vi "FOC Algorithm.vi"() -> ()   [LabVIEW 2025]
panel:
  in  "Speed Setpoint":fxp<+/-,32,16>=500.0
  in  "Kp (speed)":fxp<+,32,8>=1.2099742889404297e-05
  in  "Ki (speed)":fxp<+,32,8>=4.76837158203125e-07
  in  "PWM  Period (T)":fxp<+,32,10>=512.0
  in  "Kp (Id)":fxp<+/-,32,4>=0.6000000014901161
  in  "Ki (Id)":fxp<+/-,32,4>=0.3999999985098839
  in  "Kp (Iq)":fxp<+/-,32,8>=0.550000011920929
  in  "Ki (Iq)":fxp<+/-,32,8>=0.30000001192092896
  out "Id":fxp<+/-,32,4> format="%.6e"
  out "Iq":fxp<+/-,32,4> format="%.6e"
  out "Va":fxp<+/-,37,17> format="%.5e"
  out "Vb":fxp<+/-,37,17> format="%.5e"
  out "Vc":fxp<+/-,37,17> format="%.5e"
  in  "1/Vdc":fxp<+/-,32,16>=512.0
  out "PWM1":fxp<+,16,16>
  out "PWM2":fxp<+,16,16>
  out "PWM3":fxp<+,16,16>
  out "Vq":fxp<+/-,37,17> format="%.5e"
  out "Vd":fxp<+/-,32,4> format="%.5e"
  out "Valpha":fxp<+/-,32,12> format="%.8g"
  out "Vbeta":fxp<+/-,32,12> format="%.8g"
  out "Speed PI Output":fxp<+,32,9> format="%.8g"
  out "Ta":fxp<+/-,37,17> format="%.8g"
  out "Tb":fxp<+/-,37,17> format="%.8g"
  out "Tc":fxp<+/-,37,17> format="%.8g"
  in  "RPM":fxp<+/-,32,16>
  in  "Ia":fxp<+/-,32,4> format="%#_8g"
  in  "Ib":fxp<+/-,32,4> format="%.8g"
  in  "Theta":fxp<+/-,32,16> format="%.8g"
  in  "stop":bool
  # "Control Inputs"
  # "Control Gains"
  # "Control Constants"
  # "Calculated Values and PWM Output"
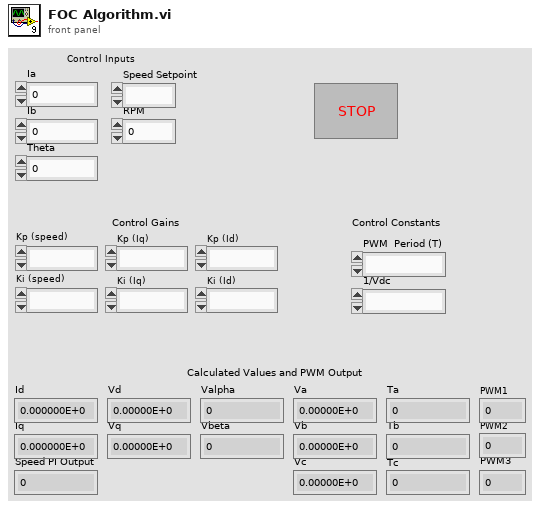
[diagram p1: front panel]
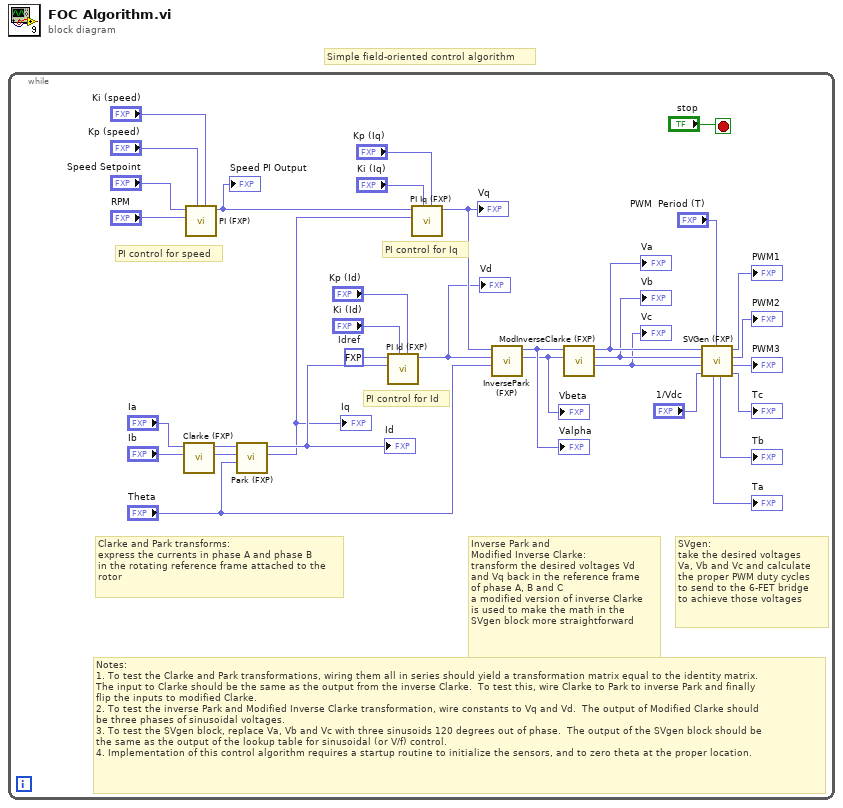
[diagram p0: block diagram]
diagram:
  # "Simple field-oriented control algorithm"
  n1 = while {
    stop <- "stop" stop-if-true
    w28 = fxp<+/-,32,1> 0.0  # Idref
    # "Notes:\n1. To test the Clarke and Park transformations, wiring them all in series should yield a transformation matrix equal to the identity matrix.\nThe input to Clarke should be the same as the output from the inverse Clarke.  To test this, wire Clarke to Park to inverse Park and finally\nflip the inputs to modified Clarke.\n2. To test the inverse Park and Modified Inverse Clarke transformation, wire constants to Vq and Vd.  The output of Modified Clarke should \nbe three phases of sinusoidal voltages.\n3. To test the SVgen block, replace Va, Vb and Vc with three sinusoids 120 degrees out of phase.  The output of the SVgen block should be\nthe same as the output of the lookup table for sinusoidal (or V/f) control.\n4. Implementation of this control algorithm requires a startup routine to initialize the sensors, and to zero theta at the proper location."
    # "SVgen:\ntake the desired voltages\nVa, Vb and Vc and calculate\nthe proper PWM duty cycles\nto send to the 6-FET bridge\nto achieve those voltages"
    # "Inverse Park and \nModified Inverse Clarke:\ntransform the desired voltages Vd\nand Vq back in the reference frame\nof phase A, B and C\na modified version of inverse Clarke\nis used to make the math in the \nSVgen block more straightforward"
    # "Clarke and Park transforms:\nexpress the currents in phase A and phase B\nin the rotating reference frame attached to the\nrotor"
    # "PI control for Id"
    # "PI control for Iq"
    # "PI control for speed"
    n2 = call "Clarke (FXP).vi"("B"="Ib", "A"="Ia") -> ("x*y"=w23:fxp<+/-,32,5>, "A"=w22:fxp<+/-,32,5>)  [unwired: 8 out]
    n3 = call "PI (FXP).vi"("Ki"="Ki (speed)", "Kp"="Kp (speed)", "Process Value"="RPM", "Setpoint"="Speed Setpoint") -> ("Output"=w7:fxp<+/-,32,12>)  [unwired: 7 out]
    "Speed PI Output" <- w7
    n4 = call "Park (FXP).vi"("Theta"="Theta", "beta"=w23, "alpha"=w22) -> (2:"x+y"=w1:fxp<+/-,32,4>, 3:"x+y"=w24:fxp<+/-,32,4>)  [unwired: 7 out]
    "Id" <- w24
    "Iq" <- w1
    n5 = call "PI Id (FXP).vi"("Process Value"="Kp (Id)", "Setpoint"="Ki (Id)", "Ki"=w24, "Kp"=w28) -> ("x+y"=w10:fxp<+/-,32,4>)  [unwired: 7 out]
    "Vd" <- w10
    n6 = call "PI Iq (FXP).vi"("Process Value"="Kp (Iq)", "Setpoint"="Ki (Iq)", "Ki"=w1, "Kp"=w7) -> ("x+y"=w25:fxp<+/-,32,12>)  [unwired: 7 out]
    "Vq" <- w25
    n7 = call "InversePark (FXP).vi"("Theta"="Theta", "d"=w10, "q"=w25) -> (2:"x+y"=w20:fxp<+/-,32,12>, 3:"x+y"=w21:fxp<+/-,32,12>)  [unwired: 7 out]
    "Valpha" <- w21
    "Vbeta" <- w20
    n8 = call "ModInverseClarke (FXP).vi"("b"=w20, "a"=w21) -> (1:"x*y"=w18:fxp<+/-,32,12>, 2:"x*y"=w19:fxp<+/-,32,12>, "b"=w26:fxp<+/-,32,12>)  [unwired: 7 out]
    "Va" <- w26
    "Vb" <- w19
    "Vc" <- w18
    n9 = call "SVGen (FXP).vi"("PWM  (Period)"="PWM  Period (T)", "1/Vdc"="1/Vdc", "Vr3"=w18, "Vr2"=w19, "Vr1"=w26) -> ("Tc"=→"Tc":fxp<+/-,37,17>, "PWM3"=→"PWM3":fxp<+,16,16>, "PWM2"=→"PWM2":fxp<+,16,16>, "PWM1"=→"PWM1":fxp<+,16,16>, 4:"x+y"=→"Tb":fxp<+/-,37,17>, 6:"x+y"=→"Ta":fxp<+/-,37,17>)  [unwired: 1 out]
  }
